vi "mul_add_18_dc_rnd.vi"(8 "add":fxp<+/-,24,16> format="%#_10g", 10 "Signal":fxp<+/-,18,16>=32.0, 11 "coeff":fxp<+/-,18,2>=0.5) -> (1 "out":fxp<+/-,24,16>)   [LabVIEW 2018]
uses:
  <vilib>/rvi/FXPMathLib/basic elements/DSP48E/simVIs/niFpgaDsp48eSimulationState.ctl
  <vilib>/rvi/FXPMathLib/basic elements/DSP48E/subVIs/niFpgaDsp48eType.ctl
  <vilib>/rvi/FXPMathLib/basic elements/DSP48E/subVIs/niFpgaDsp48eAlumodeOpmodeCarryinselState.ctl
  <vilib>/rvi/FXPMathLib/basic elements/DSP48E/subVIs/niFpgaDsp48eUseMultiplierState.ctl
  <vilib>/rvi/FXPMathLib/basic elements/DSP48E/subVIs/niFpgaDsp48eLogicUnitModeState.ctl
  <vilib>/rvi/FXPMathLib/basic elements/DSP48E/subVIs/niFpgaDsp48eSelectPatternState.ctl
  <vilib>/rvi/FXPMathLib/basic elements/DSP48E/subVIs/niFpgaDsp48eSelectMaskState.ctl
  <vilib>/rvi/FXPMathLib/basic elements/DSP48E/subVIs/niFpgaDsp48eAutoresetState.ctl
  <vilib>/rvi/FXPMathLib/basic elements/DSP48E/simVIs/niFpgaDsp48eResets.ctl
  <vilib>/rvi/FXPMathLib/basic elements/DSP48E/simVIs/niFpgaDsp48eRegisters.ctl
  <vilib>/rvi/FXPMathLib/basic elements/DSP48E/simVIs/niFpgaDsp48eCheckMode.vi
  <vilib>/rvi/FXPMathLib/basic elements/DSP48E/simVIs/niFpgaDsp48eReportInvalidMode.vi
  <vilib>/rvi/FXPMathLib/basic elements/DSP48E/simVIs/niFpgaDsp48eSimBundleEnables.vi
  <vilib>/rvi/FXPMathLib/basic elements/DSP48E/simVIs/niFpgaDsp48eSimMultiplier.vi
  <vilib>/rvi/FXPMathLib/basic elements/DSP48E/simVIs/niFpgaDsp48eSimArithmetic.vi
  <vilib>/rvi/FXPMathLib/basic elements/DSP48E/simVIs/niFpgaDsp48eSimPatternDetect.vi
  <vilib>/rvi/FXPMathLib/basic elements/DSP48E/simVIs/niFpgaDsp48eSimP.vi
  <vilib>/rvi/FXPMathLib/basic elements/DSP48E/simVIs/niFpgaDsp48eSimUpdateState.vi
  <vilib>/rvi/FXPMathLib/basic elements/DSP48E/XNode/niFpgaDsp48e.xnode
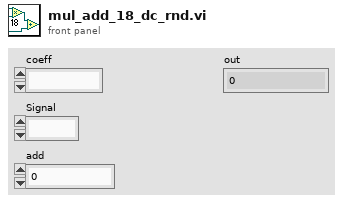
[diagram p1: front panel]
types:
  T1 = cluster{"Boolean array[0]":bool, "Boolean array[1]":bool, "Boolean array[2]":bool, "Boolean array[3]":bool, "Boolean array[4]":bool, "Boolean array[5]":bool, "Boolean array[6]":bool, "Boolean array[7]":bool, "Boolean array[8]":bool, "Boolean array[9]":bool, "Boolean array[10]":bool, "Boolean array[11]":bool, "Boolean array[12]":bool, "Boolean array[13]":bool, "Boolean array[14]":bool, "Boolean array[15]":bool, "Boolean array[16]":bool, "Boolean array[17]":bool}
  T2 = cluster{"Boolean array[0]":bool, "Boolean array[1]":bool, "Boolean array[2]":bool, "Boolean array[3]":bool, "Boolean array[4]":bool, "Boolean array[5]":bool, "Boolean array[6]":bool, "Boolean array[7]":bool, "Boolean array[8]":bool, "Boolean array[9]":bool, "Boolean array[10]":bool, "Boolean array[11]":bool, "Boolean array[12]":bool, "Boolean array[13]":bool, "Boolean array[14]":bool, "Boolean array[15]":bool, "Boolean array[16]":bool, "Boolean array[17]":bool, "Boolean array[18]":bool, "Boolean array[19]":bool, "Boolean array[20]":bool, "Boolean array[21]":bool, "Boolean array[22]":bool, "Boolean array[23]":bool}
  T3 = cluster{"Boolean array[0]":bool, "Boolean array[1]":bool, "Boolean array[2]":bool, "Boolean array[3]":bool, "Boolean array[4]":bool, "Boolean array[5]":bool, "Boolean array[6]":bool, "Boolean array[7]":bool, "Boolean array[8]":bool, "Boolean array[9]":bool, "Boolean array[10]":bool, "Boolean array[11]":bool, "Boolean array[12]":bool, "Boolean array[13]":bool, "Boolean array[14]":bool, "Boolean array[15]":bool, "Boolean array[16]":bool, "Boolean array[17]":bool, "Boolean array[18]":bool, "Boolean array[19]":bool, "Boolean array[20]":bool, "Boolean array[21]":bool, "Boolean array[22]":bool, "Boolean array[23]":bool, "Boolean array[24]":bool, "Boolean array[25]":bool, "Boolean array[26]":bool, "Boolean array[27]":bool, "Boolean array[28]":bool, "Boolean array[29]":bool, "Boolean array[30]":bool, "Boolean array[31]":bool, "Boolean array[32]":bool, "Boolean array[33]":bool, "Boolean array[34]":bool, "Boolean array[35]":bool, "Boolean array[36]":bool, "Boolean array[37]":bool, "Boolean array[38]":bool, "Boolean array[39]":bool, "Boolean array[40]":bool, "Boolean array[41]":bool, "Boolean array[42]":bool, "Boolean array[43]":bool, "Boolean array[44]":bool, "Boolean array[45]":bool, "Boolean array[46]":bool, "Boolean array[47]":bool}
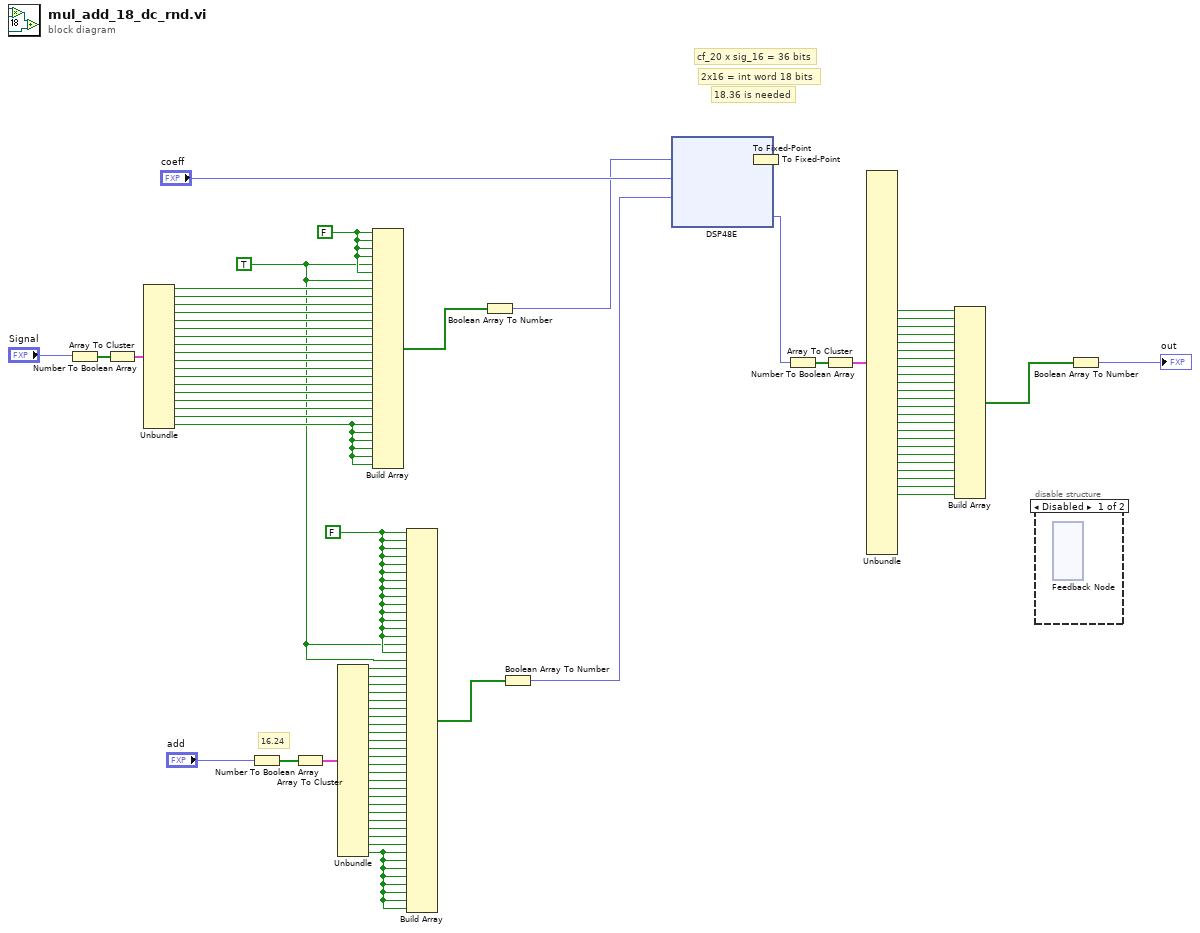
[diagram p0: block diagram]
diagram:
  w3 = TRUE ("Boolean array[0]")
  w5 = FALSE ("Boolean array[0]")
  w4 = FALSE ("Boolean array[0]")
  # "16.24"
  # "18.36 is needed"
  # "2x16 = int word 18 bits"
  # "cf_20 x sig_16 = 36 bits"
  n1 = Number To Boolean Array(number="Signal") -> (Boolean array=w38:bool[])
  n2 = Array To Cluster(array=w38) -> (cluster=w31:T1)
  n3 = Unbundle(w31) -> ("Boolean array[0]"=w14:bool, "Boolean array[1]"=w15:bool, "Boolean array[2]"=w16:bool, "Boolean array[3]"=w17:bool, "Boolean array[4]"=w18:bool, "Boolean array[5]"=w19:bool, "Boolean array[6]"=w20:bool, "Boolean array[7]"=w21:bool, "Boolean array[8]"=w22:bool, "Boolean array[9]"=w23:bool, "Boolean array[10]"=w24:bool, "Boolean array[11]"=w25:bool, "Boolean array[12]"=w26:bool, "Boolean array[13]"=w27:bool, "Boolean array[14]"=w28:bool, "Boolean array[15]"=w29:bool, "Boolean array[16]"=w30:bool, "Boolean array[17]"=w11:bool)
  n4 = Number To Boolean Array(number="add") -> (Boolean array=w86:bool[])
  n5 = Array To Cluster(array=w86) -> (cluster=w85:T2)
  n6 = Unbundle(w85) -> ("Boolean array[0]"=w62:bool, "Boolean array[1]"=w63:bool, "Boolean array[2]"=w64:bool, "Boolean array[3]"=w65:bool, "Boolean array[4]"=w66:bool, "Boolean array[5]"=w67:bool, "Boolean array[6]"=w68:bool, "Boolean array[7]"=w69:bool, "Boolean array[8]"=w70:bool, "Boolean array[9]"=w71:bool, "Boolean array[10]"=w72:bool, "Boolean array[11]"=w73:bool, "Boolean array[12]"=w74:bool, "Boolean array[13]"=w75:bool, "Boolean array[14]"=w76:bool, "Boolean array[15]"=w77:bool, "Boolean array[16]"=w78:bool, "Boolean array[17]"=w79:bool, "Boolean array[18]"=w80:bool, "Boolean array[19]"=w81:bool, "Boolean array[20]"=w82:bool, "Boolean array[21]"=w83:bool, "Boolean array[22]"=w84:bool, "Boolean array[23]"=w12:bool)
  n7 = Build Array(w5, w5, w5, w5, w3, w5, w3, w14, w15, w16, w17, w18, w19, w20, w21, w22, w23, w24, w25, w26, w27, w28, w29, w30, w11, w11, w11, w11, w11, w11) -> (w43:bool[])
  n8 = Build Array(w4, w4, w4, w4, w4, w4, w4, w4, w4, w4, w4, w4, w4, w4, w3, w4, w3, w62, w63, w64, w65, w66, w67, w68, w69, w70, w71, w72, w73, w74, w75, w76, w77, w78, w79, w80, w81, w82, w83, w84, w12, w12, w12, w12, w12, w12, w12, w12) -> (w42:bool[])
  n9 = Boolean Array To Number(Boolean array=w43) -> (number=w36:fxp<+/-,30,22>)
  n10 = Boolean Array To Number(Boolean array=w42) -> (number=w87:fxp<+/-,48,18>)
  n11 = To Fixed-Point(number=w36) -> (fixed-point=w1:fxp<+/-,30,22>)  [unwired: 1 in]
  n12 = To Fixed-Point(number=w1) -> (fixed-point=w2:fxp<+/-,25,17>)  [unwired: 1 in]
  n13 = xnode ("DSP48E")("a"=w2, "b"="coeff", "c"=w87) -> ("p"=w50:fxp<+/-,48,16>)
  n14 = Number To Boolean Array(number=w50) -> (Boolean array=w39:bool[])
  n15 = Array To Cluster(array=w39) -> (cluster=w61:T3)
  n16 = Unbundle(w61) -> ("Boolean array[17]"=w6:bool, "Boolean array[18]"=w7:bool, "Boolean array[19]"=w8:bool, "Boolean array[20]"=w9:bool, "Boolean array[21]"=w10:bool, "Boolean array[22]"=w35:bool, "Boolean array[23]"=w34:bool, "Boolean array[24]"=w54:bool, "Boolean array[25]"=w55:bool, "Boolean array[26]"=w56:bool, "Boolean array[27]"=w57:bool, "Boolean array[28]"=w58:bool, "Boolean array[29]"=w59:bool, "Boolean array[30]"=w60:bool, "Boolean array[31]"=w51:bool, "Boolean array[32]"=w52:bool, "Boolean array[33]"=w53:bool, "Boolean array[34]"=w49:bool, "Boolean array[35]"=w48:bool, "Boolean array[36]"=w41:bool, "Boolean array[37]"=w40:bool, "Boolean array[38]"=w32:bool, "Boolean array[39]"=w33:bool, "Boolean array[40]"=w13:bool)  [unwired: 24 out]
  n17 = Build Array(w6, w7, w8, w9, w10, w35, w34, w54, w55, w56, w57, w58, w59, w60, w51, w52, w53, w49, w48, w41, w40, w32, w33, w13) -> (w47:bool[])
  n18 = disable-structure shown="Disabled" {
    frame Disabled {
      n19 = feedback #1() -> ()  [unwired: 2 in]
      n20 = feedback-in #1() -> ()  [unwired: 1 in, 1 out]
    }
    frame Enabled {
    }
  }
  n21 = Boolean Array To Number(Boolean array=w47) -> (number=→"out":fxp<+/-,24,16>)
